vi "rszvl Reset.vi"(0 "VISA resource name":refnum<visa-resource-name>, 11 "error in (no error)":errorcluster) -> (4 "VISA resource name out":refnum<visa-resource-name>, 15 "error out":errorcluster)   [LabVIEW 2014]
doc: "This VI resets the instrument, and then sends a set of default setup commands to the instrument.\n\nRemote-control command(s):\n*RST\n*CLS"
uses:
  rszvl_rsidr_core.lvlib
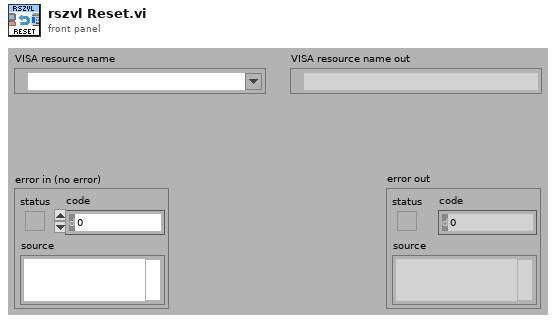
[diagram p1: front panel]
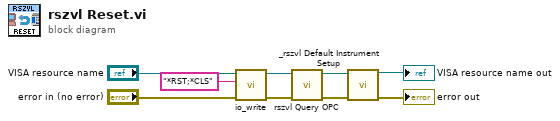
[diagram p0: block diagram]
diagram:
  n1 = call "io_write.vi"("error in"="error in (no error)", "write buffer"="*RST;*CLS" ("Reset Command"), "VISA resource name"="VISA resource name") -> ("error out"=w5:errorcluster, "VISA resource name out"=w4:refnum<visa-resource-name>)  [unwired: 7 in]
  n2 = call "rszvl Query OPC.vi"("error in (no error)"=w5, "VISA resource name"=w4) -> ("error out"=w3:errorcluster, "VISA resource name out"=w2:refnum<visa-resource-name>)  [unwired: 7 in, 1 out]
  n3 = call "_rszvl Default Instrument Setup.vi"("VISA resource name"=w2, "error in (no error)"=w3) -> ("VISA resource name out"=→"VISA resource name out":refnum<visa-resource-name>, "error out"=→"error out":errorcluster)  [unwired: 12 in]
